vi "Pre-lim Current Detection.vi"(6 "Barcodes in":string[](array[string]), 8 "error in (no error)":errorcluster, 10 "Stop Program":bool, 11 "BoardHandle in":T1) -> (0 "error out":errorcluster, 1 "channel 4 currents":dbl[](array[numeric]), 2 "channel 3 currents":dbl[](array[numeric]), 3 "channel 2 currents":dbl[](array[numeric]), 4 "BoardHandle out 3":T1, 5 "channel 1 currents":dbl[](array[numeric]), 7 "Power Supply Trip":bool, 9 "Actual Voltage Level (V)":dbl format="%#_13g")   [LabVIEW 2020]
uses:
  Program Files/National Instruments/LabVIEW 2018/instr.lib/CAEN PSM/CAEN PSM.lvlib
panel:
  out "Actual Current Limit (nA) 4":dbl format="%#_13g"
  out "Actual Current Limit (nA) 3":dbl format="%#_13g"
  out "Actual Current Limit (nA) 2":dbl format="%#_13g"
  out "Actual Current Limit (nA)":dbl format="%#_13g"
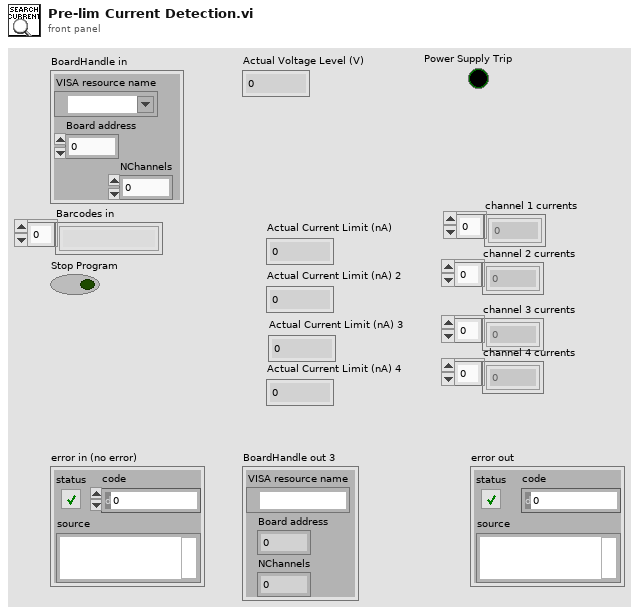
[diagram p1: front panel]
types:
  T1 = cluster{"VISA resource name":refnum<visa-resource-name>, "Board address":u8, "NChannels":u8}
  T2 = typedef "CAEN PSM.lvlib/BoardHandle.ctl" = cluster{"VISA resource name":refnum<visa-resource-name>, "Board address":u8, "NChannels":u8}
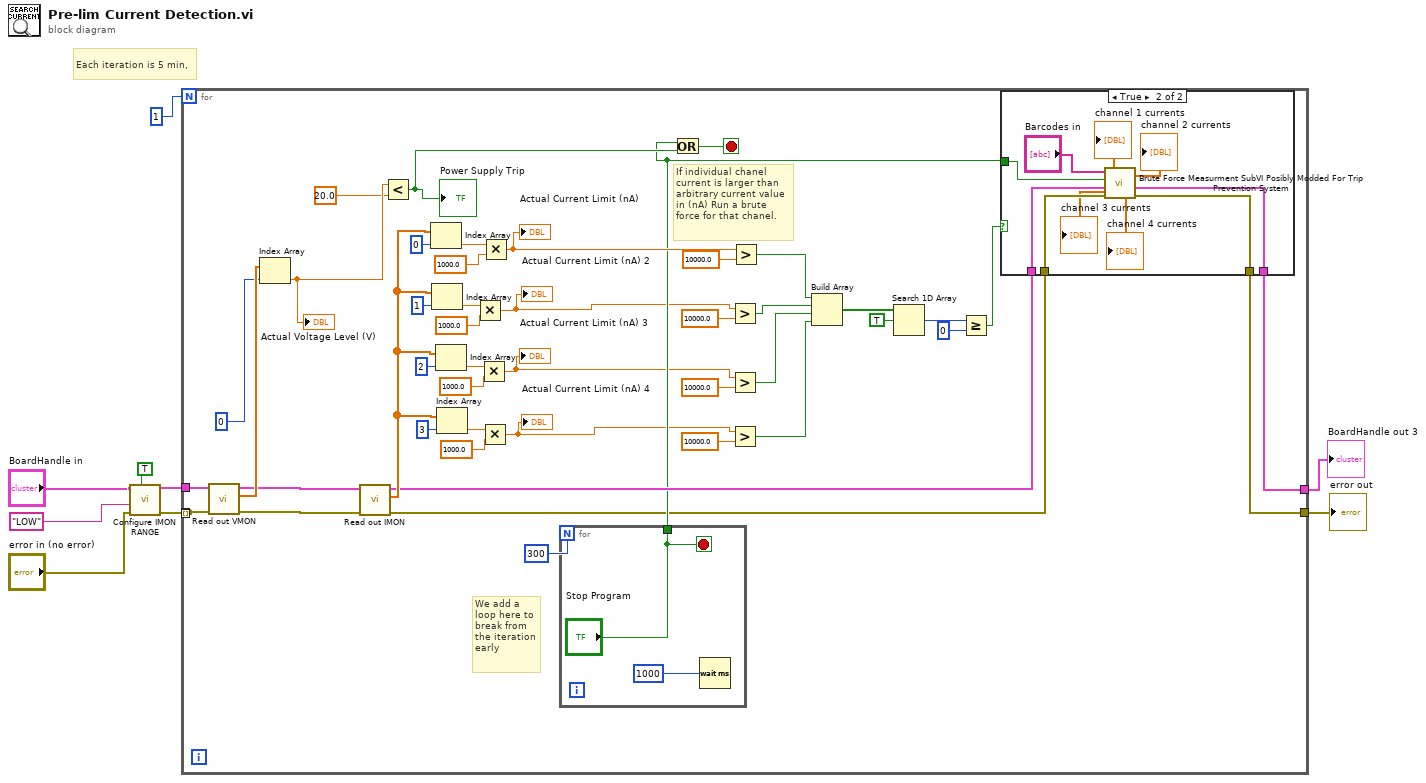
[diagram p0: block diagram]
diagram:
  # "Each iteration is 5 min,"
  n1 = call "Configure IMON RANGE.vi"("All Channels (F)"=TRUE, "error in (no error)"="error in (no error)", "IMon range (LOW)"="LOW", "BoardHandle"="BoardHandle in") -> ("error out"=w6:errorcluster, "BoardHandle out"=w5:T2)  [unwired: 6 in]
  n2 = for {
    N: 1 ("N") -> [_]
    tunnel: w6 -> [w45]
    tunnel: [w26] -> w2
    tunnel: [w25] -> w1
    tunnel: w5 -> [w46]
    tunnel: [w45] -> _ mode=indexing
    stop <- w49 stop-if-true
    # "If individual chanel\ncurrent is larger than\narbitrary current value\nin (nA) Run a brute \nforce for that chanel."
    # "We add a \nloop here to\nbreak from \nthe iteration\nearly"
    n3 = call "Read out VMON.vi"("error in (no error)"=w45, "BoardHandle"=w46) -> ("error out"=w53:errorcluster, "VMon values (V)"=w55:dbl[], "BoardHandle out"=w54:T2)  [unwired: 7 in]
    n4 = Index Array(array=w55, index=0) -> (element=w51:dbl)
    "Actual Voltage Level (V)" <- w51
    n5 = call "Read out IMON.vi"("error in (no error)"=w53, "BoardHandle"=w54) -> ("error out"=w27:errorcluster, "IMon values (uA)"=w33:dbl[], "BoardHandle out"=w29:T2)  [unwired: 6 in, 1 out]
    n6 = Less?(x=w51, y=20.0) -> (x < y?=w48:bool)
    "Power Supply Trip" <- w48
    n7 = Index Array(array=w33, index=0) -> (element=w32:dbl)
    n8 = Index Array(array=w33, index=1) -> (element=w42:dbl)
    n9 = Index Array(array=w33, index=2) -> (element=w39:dbl)
    n10 = Index Array(array=w33, index=3) -> (element=w36:dbl)
    n11 = Multiply(x=w42, y=1000.0) -> (x*y=w21:dbl)
    "Actual Current Limit (nA) 2" <- w21
    n12 = Multiply(x=w39, y=1000.0) -> (x*y=w20:dbl)
    "Actual Current Limit (nA) 3" <- w20
    n13 = Multiply(x=w36, y=1000.0) -> (x*y=w19:dbl)
    "Actual Current Limit (nA) 4" <- w19
    n14 = Multiply(x=w32, y=1000.0) -> (x*y=w31:dbl)
    "Actual Current Limit (nA)" <- w31
    n15 = for {
      N: 300 ("dt (s) in") -> [_]
      tunnel: ["Stop Program"] -> w28
      stop <- "Stop Program" stop-if-true
      n16 = Wait (ms)(milliseconds to wait=1000) -> ()  [unwired: 1 out]
    }
    n17 = Or(x=w28, y=w48) -> (x .or. y?=w49:bool)
    n18 = Greater?(x=w21, y=10000.0) -> (0:w17:bool)
    n19 = Greater?(x=w20, y=10000.0) -> (0:w16:bool)
    n20 = Greater?(x=w19, y=10000.0) -> (0:w15:bool)
    n21 = Greater?(x=w31, y=10000.0) -> (0:w18:bool)
    n22 = Build Array(w18, w17, w16, w15) -> (w14:bool[])
    n23 = Search 1D Array(1D array=w14, element=TRUE) -> (index of element=w12:i32)  [unwired: 1 in]
    n24 = Greater Or Equal?(x=w12, y=0) -> (x >= y?=w10:bool)
    n25 = case shown="True" w10 {
      tunnel: w29 -> [w56 w66]
      tunnel: w28 -> [_ w65]
      tunnel: w27 -> [w57 w64]
      tunnel: [w56 w63] -> w26
      tunnel: [w57 w62] -> w25
      frame False {
      }
      frame True {
        n26 = call "Brute Force Measurment SubVI Posibly Modded For Trip Prevention System.vi"("error in (no error)"=w64, "BoardHandle in"=w66, "Stop Program Brute Force"=w65, "Barcodes in"="Barcodes in") -> ("error out"=w62:errorcluster, "BoardHandle out"=w63:T1, "channel 4 currents"=→"channel 4 currents":dbl[], "channel 2 currents"=→"channel 2 currents":dbl[], "channel 3 currents"=→"channel 3 currents":dbl[], "channel 1 currents"=→"channel 1 currents":dbl[])  [unwired: 1 in, 1 out]
      }
    }
  }
  "error out" <- w1
  "BoardHandle out 3" <- w2
